vi "dmmmmmmtolatlon.vi"(2 "Longitude  dmm.mmmmm":ext format="%#_13g", 3 "Latitude  dmm.mmmmm":ext format="%#_13g") -> (0 "Longitude":dbl format="%#_16g", 1 "Latitude":dbl format="%#_16g")   [LabVIEW 2010]
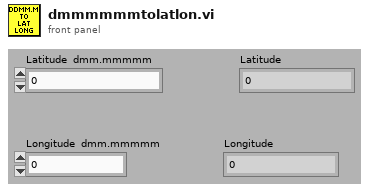
[diagram p1: front panel]
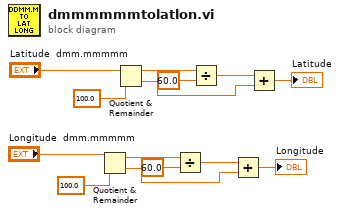
[diagram p0: block diagram]
diagram:
  n1 = Quotient & Remainder(x="Longitude  dmm.mmmmm", y=100.0) -> (x-y*floor(x/y)=w3:ext, floor(x/y)=w6:ext)
  n2 = Quotient & Remainder(x="Latitude  dmm.mmmmm", y=100.0) -> (x-y*floor(x/y)=w12:ext, floor(x/y)=w9:ext)
  n3 = Divide(x=w3, y=60.0) -> (x/y=w5:ext)
  n4 = Divide(x=w12, y=60.0) -> (x/y=w10:ext)
  n5 = Add(x=w5, y=w6) -> (x+y=→"Longitude":ext)
  n6 = Add(x=w10, y=w9) -> (x+y=→"Latitude":ext)
